vi "KepcoDCPwr Current List Example.vi"(0 "VISA resource name":refnum<visa-resource-name>, 11 "error in (no error)":errorcluster) -> (15 "error out":errorcluster)   [LabVIEW 2013]
doc: "Current list example\n\nSends a list of points to power supply consiting of current oputput settings.\n\nVoltage is set ot value indicated by VI \n\nList is executed."
panel:
  out "Instrument Error":errorcluster
  in  "Start":bool
  in  "Exit":bool
  in  "Voltage":dbl format="%.2f"
  out "Voltage vs Time":cluster{dbl[], dbl[]}(graph)
  in  "Stop":bool
  in  "Disable @ End":bool
  in  "# of Cycles":i32=1
  in  "Current Increment":dbl format="%.2f"
  in  "Dwell (sec)":dbl format="%.4f"
  in  "End (Current)":dbl format="%.2f"
  in  "Start (Current)":dbl format="%.2f"
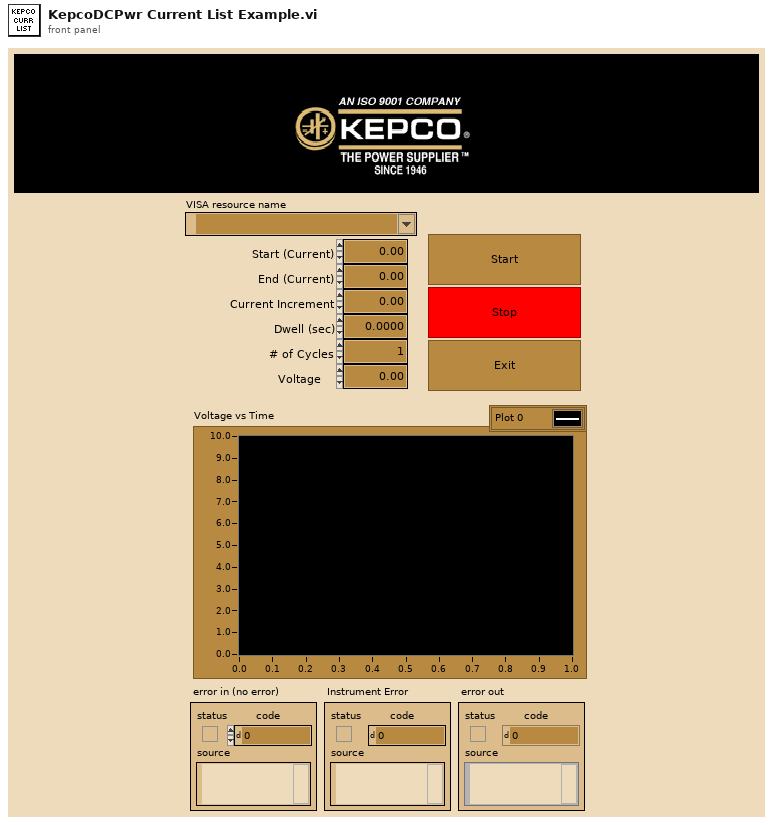
[diagram p1: front panel]
types:
  T1 = cluster{bool, "error code":i32, "error message":string}
  T2 = enum16{"Fixed", "List", "Transient", "External", "Gain", "Protect", "Additive"}
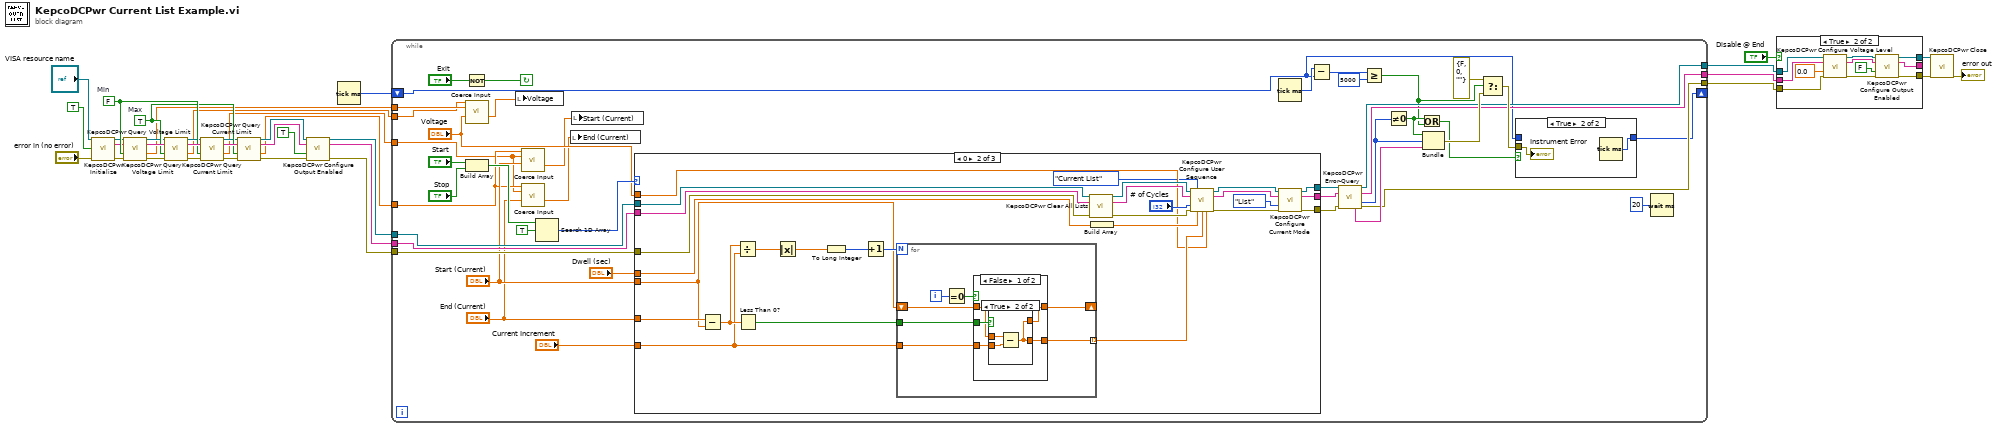
[diagram p0: block diagram]
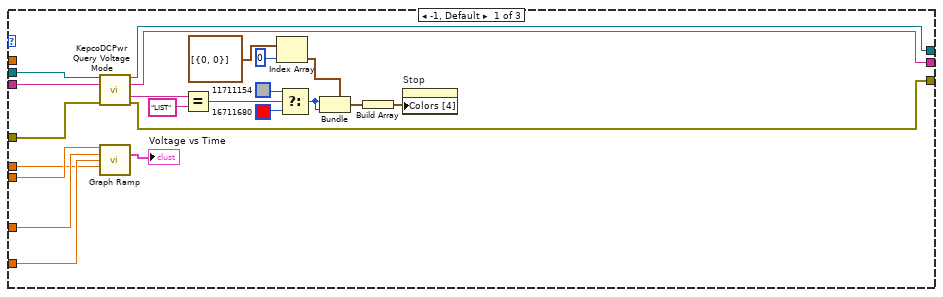
[diagram p3: hidden frame]
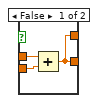
[diagram p4: hidden frame]
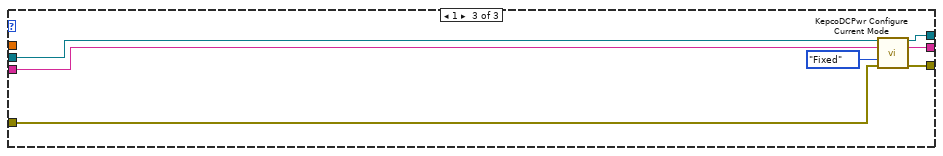
[diagram p6: hidden frame]
diagram:
  w16 = TRUE  # Max
  w17 = FALSE  # Min
  n1 = call "KepcoDCPwr Initialize.vi"("VISA Resource Name"="VISA resource name", "id query (True)"=TRUE, "error in (no error)"="error in (no error)") -> ("VISA Session Out"=w7:refnum<visa-resource-name>, "Model Out"=w9:string, "error out"=w11:errorcluster)  [unwired: 3 in, 7 out]
  n2 = call "KepcoDCPwr Query Voltage Limit.vi"("VISA Session"=w7, "Model In"=w9, "Max Level (T),MIN LEVEL(F)"=w17, "error in (no error)"=w11) -> ("VISA Session Out"=w13:refnum<visa-resource-name>, "Model Out"=w22:string, "voltage level"=w1:dbl, "error out"=w23:errorcluster)  [unwired: 1 in, 7 out]
  n3 = call "KepcoDCPwr Query Voltage Limit.vi"("VISA Session"=w13, "Model In"=w22, "Max Level (T),MIN LEVEL(F)"=w16, "error in (no error)"=w23) -> ("VISA Session Out"=w14:refnum<visa-resource-name>, "Model Out"=w18:string, "voltage level"=w2:dbl, "error out"=w21:errorcluster)  [unwired: 1 in, 7 out]
  n4 = call "KepcoDCPwr Query Current Limit.vi"("VISA Session"=w14, "Model In"=w18, "Level"=w17, "error in (no error)"=w21) -> ("VISA Session Out"=w15:refnum<visa-resource-name>, "Model Out"=w19:string, "current limit"=w4:dbl, "error out"=w20:errorcluster)  [unwired: 1 in, 7 out]
  n5 = call "KepcoDCPwr Query Current Limit.vi"("VISA Session"=w15, "Model In"=w19, "Level"=w16, "error in (no error)"=w20) -> ("VISA Session Out"=w8:refnum<visa-resource-name>, "Model Out"=w10:string, "current limit"=w3:dbl, "error out"=w12:errorcluster)  [unwired: 1 in, 7 out]
  n6 = call "KepcoDCPwr Configure Output Enabled.vi"("VISA Session"=w8, "Model In"=w10, "Input enabled (True)"=TRUE, "error in (no error)"=w12) -> ("VISA Session Out"=w32:refnum<visa-resource-name>, "Model Out"=w31:string, "error out"=w30:errorcluster)  [unwired: 9 out]
  n7 = Tick Count (ms)() -> (millisecond timer value=w6:u32)
  n8 = while {
    shift-left: w6 -> [w39]
    shift-right: [w38] -> _
    tunnel: w2 -> [w63]
    tunnel: w1 -> [w64]
    tunnel: w3 -> [w58]
    tunnel: w4 -> [w57]
    tunnel: [w42] -> w27
    tunnel: [w40] -> w28
    tunnel: [w44] -> w29
    tunnel: w32 -> [w78]
    tunnel: w31 -> [w77]
    tunnel: w30 -> [w76]
    stop <- w75 continue-if-true
    n9 = Not(x="Exit") -> (.not. x?=w75:bool)
    n10 = call "Coerce Input.vi"("Max"=w63, "Min"=w64, "Input"="Voltage") -> ("Output"=w65:dbl)  [unwired: 12 out]
    n11 = Build Array("Start", "Stop") -> (w72:bool[])
    n12 = local write "Voltage"(w65) -> ()
    n13 = call "Coerce Input.vi"("Max"=w58, "Min"=w57, "Input"="Start (Current)") -> ("Output"=w61:dbl)  [unwired: 12 out]
    n14 = call "Coerce Input.vi"("Max"=w58, "Min"=w57, "Input"="End (Current)") -> ("Output"=w59:dbl)  [unwired: 12 out]
    n15 = Search 1D Array(1D array=w72, element=TRUE) -> (index of element=w71:i32)  [unwired: 1 in]
    n16 = local write "End (Current)"(w59) -> ()
    n17 = local write "Start (Current)"(w61) -> ()
    n18 = case shown="0" w71 {
      tunnel: w78 -> [w98 w122 w153]
      tunnel: w77 -> [w96 w121 w155]
      tunnel: w76 -> [w94 w120 w157]
      tunnel: [w97 w117 w152] -> w45
      tunnel: [w95 w113 w154] -> w41
      tunnel: [w93 w112 w156] -> w43
      tunnel: "Current Increment" -> [w100 w111 _]
      tunnel: "End (Current)" -> [w101 w110 _]
      tunnel: "Start (Current)" -> [w102 w109 _]
      tunnel: "Dwell (sec)" -> [w99 w108 _]
      tunnel: "Voltage" -> [_ w106 _]
      frame -1, Default {
        n19 = call "KepcoDCPwr Query Voltage Mode.vi"("VISA Session"=w98, "Model In"=w96, "error in (no error)"=w94) -> ("VISA Session Out"=w97:refnum<visa-resource-name>, "Model Out"=w95:string, "Mode"=w89:string, "error out"=w93:errorcluster)  [unwired: 1 in, 8 out]
        n20 = call "Graph Ramp.vi"("Start (Volts)"=w102, "End (volts)"=w101, "Voltage Increment"=w100, "Dwell (sec)"=w99) -> ("Voltage vs Time"=→"Voltage vs Time":cluster{dbl[], dbl[]})  [unwired: 11 out]
        n21 = Equal?(x=w89, y="LIST") -> (x = y?=w87:bool)
        n22 = Index Array(array=cluster{u32, u32}[] [{0, 0}] ("Colors [4]"), index=0) -> (element=w91:cluster{u32, u32})
        n23 = Select(t=u32 11711154, s=w87, f=u32 16711680) -> (s? t:f=w84:u32)
        n24 = Bundle(cluster=w91, w84, w84) -> (w90:cluster{u32, u32})
        n25 = Build Array(w90) -> (w82:cluster{u32, u32}[])
        n26 = property on="Stop" class="Bool"("Colors [4]"=w82) -> ()  [unwired: 2 in, 2 out]
      }
      frame 0 {
        n27 = Subtract(x=w110, y=w109) -> (x-y=w128:dbl)
        n28 = Divide(x=w128, y=w111) -> (x/y=w125:dbl)
        n29 = Less Than 0?(x=w128) -> (x < 0?=w130:bool)
        n30 = Absolute Value(x=w125) -> (abs(x)=w126:dbl)
        n31 = To Long Integer(number=w126) -> (32bit integer=w127:i32)
        n32 = Increment(x=w127) -> (x+1=w129:i32)
        n33 = for {
          N: w129 -> [_]
          tunnel: w130 -> [w138]
          tunnel: w111 -> [w136]
          shift-right: [w135] -> _
          shift-left: w109 -> [w137]
          tunnel: [w134] -> w107 mode=indexing
          i -> [w133]
          n34 = Equal To 0?(x=w133) -> (x = 0?=w132:bool)
          n35 = case shown="False" w132 {
            tunnel: w138 -> [w143 _]
            tunnel: w137 -> [w142 w150]
            tunnel: w136 -> [w141 _]
            tunnel: [w140 w150] -> w135
            tunnel: [w139 w150] -> w134
            frame False {
              n36 = case shown="True" w143 {
                tunnel: [w144 w147] -> w139
                tunnel: w142 -> [w146 w148]
                tunnel: w141 -> [w145 w149]
                tunnel: [w144 w147] -> w140
                frame False {
                  n37 = Add(x=w146, y=w145) -> (x+y=w144:dbl)
                }
                frame True {
                  n38 = Subtract(x=w148, y=w149) -> (x-y=w147:dbl)
                }
              }
            }
            frame True {
            }
          }
        }
        n39 = call "KepcoDCPwr Clear All Lists.vi"("VISA Session"=w122, "Model In"=w121, "error in (no error)"=w120) -> ("VISA Session Out"=w123:refnum<visa-resource-name>, "Model Out"=w118:string, "error out"=w119:errorcluster)  [unwired: 1 in, 9 out]
        n40 = Build Array(w108) -> (w124:dbl[])
        n41 = call "KepcoDCPwr Configure User Sequence.vi"("VISA Session"=w123, "List Mode (volt/current)"=enum16{"Current List", "Voltage List"}."Current List" ("List Type (DWell)"), "Model In"=w118, "# of Cycles"="# of Cycles", "error in (no error)"=w119, "Dwell (sec)"=w124, "List Data"=w107, "Limit Value"=w106) -> ("VISA Session Out"=w116:refnum<visa-resource-name>, "Model Out"=w114:string, "error out"=w115:errorcluster)  [unwired: 1 in, 4 out]
        n42 = call "KepcoDCPwr Configure Current Mode.vi"("VISA Session"=w116, "Model In"=w114, "Mode (Fixed)"=T2."List", "error in (no error)"=w115) -> ("VISA Session Out"=w117:refnum<visa-resource-name>, "Model Out"=w113:string, "error out"=w112:errorcluster)  [unwired: 8 in, 1 out]
      }
      frame 1 {
        n43 = call "KepcoDCPwr Configure Current Mode.vi"("VISA Session"=w153, "Model In"=w155, "Mode (Fixed)"=T2."Fixed", "error in (no error)"=w157) -> ("VISA Session Out"=w152:refnum<visa-resource-name>, "Model Out"=w154:string, "error out"=w156:errorcluster)  [unwired: 8 in, 1 out]
      }
    }
    n44 = Tick Count (ms)() -> (millisecond timer value=w55:u32)
    n45 = Subtract(x=w55, y=w39) -> (x-y=w54:u32)
    n46 = call "KepcoDCPwr Error-Query.vi"("VISA Session"=w45, "Model In"=w41, "error in (no error)"=w43) -> ("VISA Session Out"=w44:refnum<visa-resource-name>, "Model Out"=w40:string, "error code"=w48:i32, "error message"=w47:string, "error out"=w42:errorcluster)  [unwired: 1 in, 7 out]
    n47 = Greater Or Equal?(x=w54, y=u32 5000) -> (x >= y?=w37:bool)
    n48 = Not Equal To 0?(x=w48) -> (x != 0?=w49:bool)
    n49 = Or(x=w49, y=w37) -> (x .or. y?=w46:bool)
    n50 = Bundle(w49, "error code"=w48, "error message"=w47) -> (w50:T1)  [unwired: 1 out]
    n51 = Select(t=T1 {FALSE, "error code"=0, "error message"=""}, s=w37, f=w50) -> (s? t:f=w51:T1)
    n52 = case shown="True" w46 {
      tunnel: [w79 w81] -> w38
      tunnel: w39 -> [w79 _]
      tunnel: w51 -> [_ w80]
      frame False {
      }
      frame True {
        n53 = Tick Count (ms)() -> (millisecond timer value=w81:u32)
        "Instrument Error" <- w80
      }
    }
    n54 = Wait (ms)(milliseconds to wait=u32 20) -> ()  [unwired: 1 out]
  }
  n55 = case shown="True" "Disable @ End" {
    tunnel: w29 -> [w160 w171]
    tunnel: w28 -> [w159 w170]
    tunnel: w27 -> [w158 w169]
    tunnel: [w158 w164] -> w35
    tunnel: [w160 w163] -> w36
    tunnel: [w159 w162] -> _
    frame False {
    }
    frame True {
      n56 = call "KepcoDCPwr Configure Voltage Level.vi"("VISA Session"=w171, "Model In"=w170, "level (0.0 volts)"=0.0, "error in (no error)"=w169) -> ("VISA Session Out"=w167:refnum<visa-resource-name>, "Model Out"=w166:string, "error out"=w165:errorcluster)  [unwired: 1 in, 8 out]
      n57 = call "KepcoDCPwr Configure Output Enabled.vi"("VISA Session"=w167, "Model In"=w166, "Input enabled (True)"=FALSE ("output enabled (True)"), "error in (no error)"=w165) -> ("VISA Session Out"=w163:refnum<visa-resource-name>, "Model Out"=w162:string, "error out"=w164:errorcluster)  [unwired: 9 out]
    }
  }
  n58 = call "KepcoDCPwr Close.vi"("VISA Session"=w36, "error in (no error)"=w35) -> ("error out"=→"error out":errorcluster)  [unwired: 13 out]
